vi "Write Scalar U16.vi"(8 "error in (no error)":errorcluster, 10 "value":u16, 11 "pointer in":u64) -> (0 "error out":errorcluster, 3 "pointer out":u64)   [LabVIEW 2013, in "Shared Memory.lvlib"]
uses:
  Shared Memory.lvlib
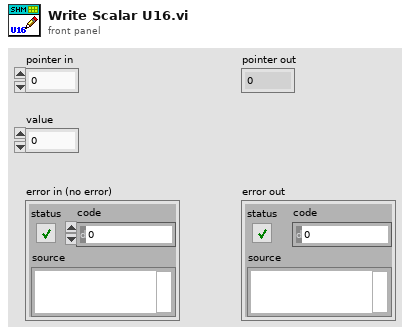
[diagram p1: front panel]
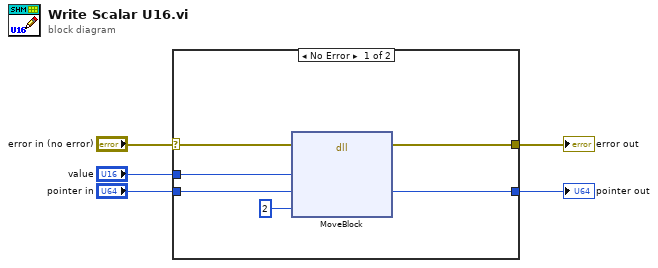
[diagram p0: block diagram]
diagram:
  n1 = case shown="No Error" "error in (no error)" {
    selector: "error in (no error)" -> [w10 w13]
    tunnel: [w9 w13] -> w5
    tunnel: "pointer in" -> [w8 w12]
    tunnel: "value" -> [w6 _]
    tunnel: [w7 w12] -> w1
    frame No Error {
      n2 = dll-call lib="LabVIEW" fn="MoveBlock"(error in=w10, "data"=w6, "pointer"=w8, "size"=u64 2) -> (error out=w9:errorcluster, "pointer"=w7:u64)  [unwired: 5 in, 1 out]
    }
    frame Error {
    }
  }
  "error out" <- w5
  "pointer out" <- w1
